vi "Initialize.vi"(8 "error in (no error)":errorcluster, 9 "settings":T1, 10 "name":string, 11 "Configuration in":refnum<class "Configuration.lvclass">) -> (0 "error out":errorcluster, 3 "Configuration out":refnum<class "Configuration.lvclass">)   [LabVIEW 2017, in "DSF Core.lvlib" / "Configuration.lvclass"]
uses:
  Configuration.lvclass
  DSF Configuration API/Public/Controls/DSF Settings Info.ctl
  Configuration.lvclass/Configuration.ctl
  DSF Core.lvlib
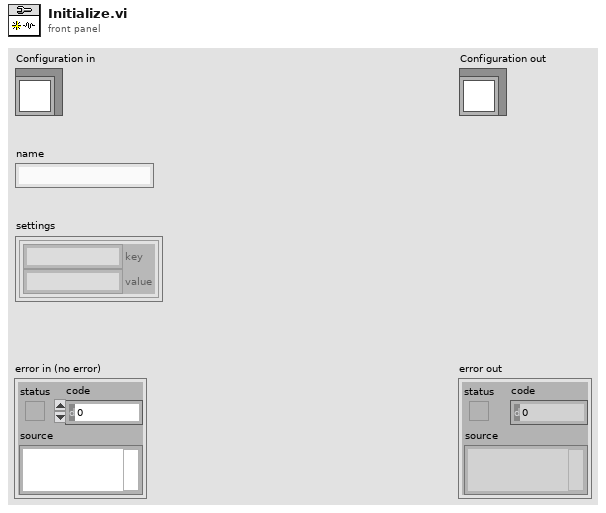
[diagram p1: front panel]
types:
  T1 = typedef "DSF Core.lvlib/DSF Settings Info.ctl" = cluster{"key":string, "value":string}[]
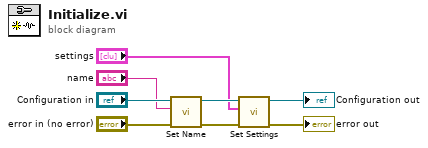
[diagram p0: block diagram]
diagram:
  n1 = call "Set Name.vi"("error in (no error)"="error in (no error)", "name"="name", "Configuration in"="Configuration in") -> ("error out"=w4:errorcluster, "Configuration out"=w7:refnum<class "Configuration.lvclass">)  [unwired: 7 in]
  n2 = call "Set Settings.vi"("error in (no error)"=w4, "settings"="settings", "Configuration in"=w7) -> ("error out"=→"error out":errorcluster, "Configuration out"=→"Configuration out":refnum<class "Configuration.lvclass">)  [unwired: 7 in]
